vi "Climber Controller.vi"(8 "error in":errorcluster) -> ()   [LabVIEW 2015]
doc: "This VI executes continuously carrying out the current operation and responding to updates or new operations. It will often contain the timing or control code that is difficult to place directly in TeleOp. This VI generally opens all sensors and motors and isolates the rest of the robot code from knowing how the operations are carried out."
uses:
  Climber Setpoints.ctl
  Climber Operations.ctl
  <vilib>/Rock Robotics/WPI/Solenoid/WPI_SolenoidChannel.ctl
  <vilib>/Rock Robotics/WPI/Solenoid/WPI_SolenoidValue.ctl
  <vilib>/Rock Robotics/WPI/Solenoid/WPI_SolenoidOpenDouble.vi
  <vilib>/Rock Robotics/WPI/Solenoid/WPI_SolenoidSetEnum.vi
  <vilib>/Rock Robotics/Network Tables/NT Write Boolean.vi
panel:
  out "Current\nCmd":string
  # "Tip: It may be helpful to observe inputs and sensor values.\nYou may also want to display tuning or debugging controls."
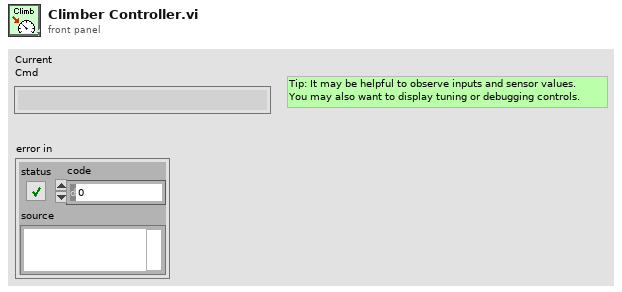
[diagram p1: front panel]
types:
  T1 = typedef "WPI_SolenoidChannel.ctl" = enum8{"Solenoid 0", "Solenoid 1", "Solenoid 2", "Solenoid 3", "Solenoid 4", "Solenoid 5", "Solenoid 6", "Solenoid 7", "Invalid"}
  T2 = typedef "Climber Setpoints.ctl" = cluster{"Operation":T3, "Setpoint":dbl, "Duration":dbl}
  T3 = typedef "Climber Operations.ctl" = enum16{"Reserve", "Read Current", "Immediate"}
  T4 = typedef "WPI_SolenoidDevRef.ctl" = cluster{"DevStatus":errorcluster, "Pneumatics Control Module":u8, "Forward Solenoid Channel":T1, "Reverse Solenoid Channel":T1}
  T5 = typedef "Command Status Info.ctl" = cluster{"Name":string, "Status":T6, "notifier out":T7}
  T6 = typedef "Completion Status.ctl" = enum16{"Successful", "Aborted", "Incomplete"}
  T7 = typedef "Completion Notifier.ctl" = refnum<notifier>
  T8 = cluster{"Default Command":T2, "Command Timing":cluster{"Start Time (ms)":u32, "Iterations":i32}, "Command Arguments":cluster{"Command Info":T5, "Description":string, "Default Command":T2, "notifier out":refnum<notifier>, "Subsystem Name":string}}
  T9 = typedef "WPI_SolenoidValue.ctl" = enum16{"Off", "On", "Forward", "Reverse"}
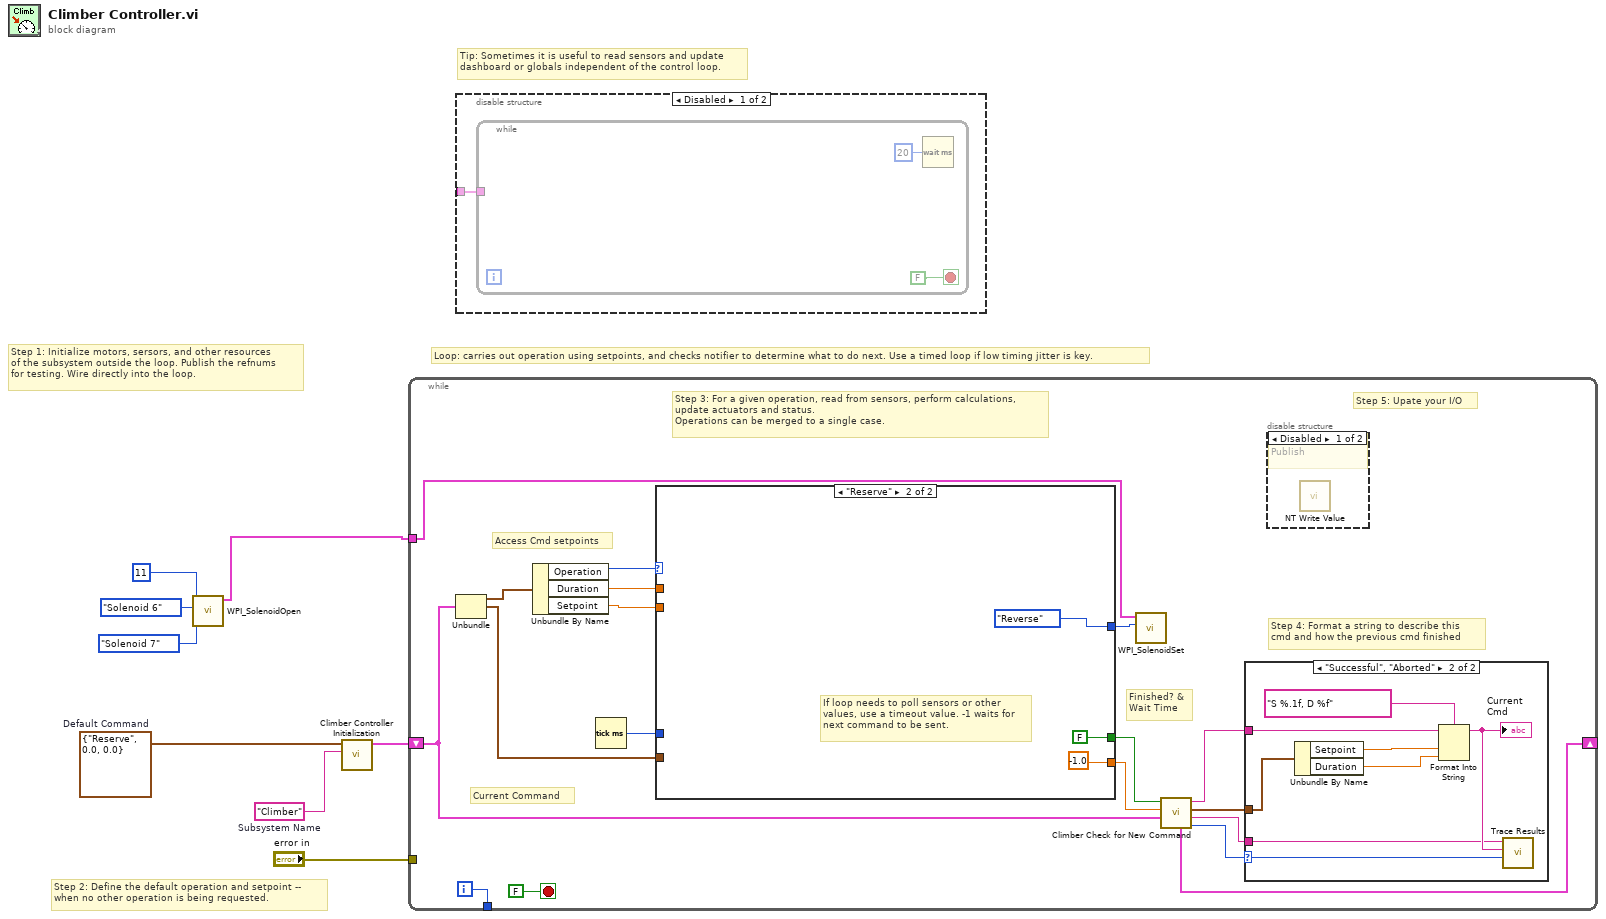
[diagram p0: block diagram]
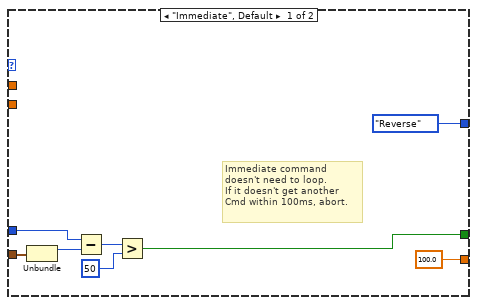
[diagram p5: hidden frame]
diagram:
  w5 = T2 {"Operation"=enum."Reserve", "Setpoint"=0.0, "Duration"=0.0}  # Default Command
  w6 = "Climber"  # Subsystem Name
  # "Tip: Sometimes it is useful to read sensors and update\ndashboard or globals independent of the control loop."
  # "Step 2: Define the default operation and setpoint --\nwhen no other operation is being requested."
  # "Step 1: Initialize motors, sersors, and other resources\nof the subsystem outside the loop. Publish the refnums\nfor testing. Wire directly into the loop."
  # "Loop: carries out operation using setpoints, and checks notifier to determine what to do next. Use a timed loop if low timing jitter is key."
  n1 = call-poly <vilib>:"WPI_SolenoidOpen.vi"("Reverse Solenoid Channel"=WPI_SolenoidChannel."Solenoid 7", "Forward Solenoid Channel"=WPI_SolenoidChannel."Solenoid 6" ("Solenoid Channel"), "Pneumatics Control Module (0)"=u8 11) -> ("SolenoidDevRef"=w1:T4)  [unwired: 7 in, 1 out]
  n2 = call "Climber Controller Initialization.vi"("Subsystem Name"=w6, "Default Command"=w5) -> ("Command Info"=w7:T8)  [unwired: 9 in]
  n3 = while {
    shift-right: [w17] -> _
    shift-left: w7 -> [w18]
    tunnel: [w25] -> _
    tunnel: "error in" -> [_]
    tunnel: w1 -> [w9]
    i -> [w25]
    stop <- FALSE stop-if-true
    # "Step 5: Upate your I/O"
    # "Step 4: Format a string to describe this\ncmd and how the previous cmd finished"
    # "Current Command"
    # "Access Cmd setpoints"
    # "Finished? &\nWait Time"
    # "Step 3: For a given operation, read from sensors, perform calculations,\nupdate actuators and status.\nOperations can be merged to a single case."
    n4 = Unbundle(w18) -> ("Default Command"=w24:T2, "Command Timing"=w20:cluster{"Start Time (ms)":u32, "Iterations":i32})  [unwired: 1 out]
    n5 = Unbundle By Name(w24) -> ("Operation"=w23:T3, "Duration"=w22:dbl, "Setpoint"=w19:dbl)
    n6 = Tick Count (ms)() -> (millisecond timer value=w21:u32)
    n7 = case shown="\"Reserve\"" w23 {
      tunnel: [100.0 -1.0] -> w15
      tunnel: [w36 FALSE ("ignore previous (F)")] -> w16
      tunnel: w20 -> [w38 _]
      tunnel: w22 -> [_ _]
      tunnel: w21 -> [w37 _]
      tunnel: w19 -> [_ _]
      tunnel: [WPI_SolenoidValue."Reverse" ("Value") WPI_SolenoidValue."Reverse" ("Value")] -> w10
      frame "Immediate", Default {
        # "Immediate command\ndoesn't need to loop.\nIf it doesn't get another\nCmd within 100ms, abort."
        n8 = Unbundle(w38) -> ("Start Time (ms)"=w41:u32)  [unwired: 1 out]
        n9 = Subtract(x=w37, y=w41) -> (x-y=w40:u32)
        n10 = Greater?(x=w40, y=u8 50 ("Left Motor")) -> (0:w36:bool)
      }
      frame "Reserve" {
        # "If loop needs to poll sensors or other\nvalues, use a timeout value. -1 waits for\nnext command to be sent."
      }
    }
    n11 = call-poly <vilib>:"WPI_SolenoidSet.vi"("Value"=w10, "SolenoidDevRef"=w9) -> ()  [unwired: 8 in, 2 out]
    n12 = call "Climber Check for New Command.vi"("Current Command"=w18, "Wait time (ms)"=w15, "Finished?"=w16) -> ("Completion"=w11:T6, "Subsystem Name"=w12:string, "Current Command"=w13:T2, "Initial Trace String"=w14:string, "NextCommand"=w17:T8)  [unwired: 4 in]
    n13 = case shown="\"Successful\", \"Aborted\"" w11 {
      selector: w11 -> [_ w34]
      tunnel: w14 -> [_ w30]
      tunnel: w13 -> [_ w31]
      tunnel: w12 -> [_ w27]
      frame "Incomplete", Default {
        # "Continuing current command"
      }
      frame "Successful", "Aborted" {
        # "Report and setup for next command"
        n14 = Unbundle By Name(w31) -> ("Setpoint"=w33:dbl, "Duration"=w28:dbl)
        n15 = Format Into String(format string="S %.1f, D %f", initial string=w30, w33, w28) -> (resulting string=w29:string)  [unwired: 1 in, 1 out]
        "Current\nCmd" <- w29
        n16 = call <vilib>:"Trace Results.vi"("Status of previous command"=w34, "Description"=w29, "Subsystem"=w27) -> ()  [unwired: 9 in]
      }
    }
    n17 = disable-structure shown="Disabled" {
      frame Disabled {
        # "Publish"
        n18 = call-poly <vilib>:"NT Write Value.vi"() -> ()  [unwired: 11 in, 1 out]
      }
      frame Enabled {
      }
    }
  }
  n19 = disable-structure shown="Disabled" {
    disable-tunnel: _ -> [w46 _]
    frame Disabled {
      n20 = while {
        tunnel: w46 -> [_]
        stop <- FALSE stop-if-true
        n21 = Wait (ms)(milliseconds to wait=u32 20) -> ()  [unwired: 1 out]
      }
    }
    frame Enabled {
    }
  }
